vi "Global 1.vi"() -> ()   [LabVIEW 2019]
panel:
  in  "Last Value":bool
  in  "count":dbl
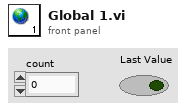
[diagram p1: front panel]
diagram:
